vi "Ball at defense area.vi"(10 "IA State":T1) -> (2 "Ball at defense area ?":bool)   [LabVIEW 2016]
uses:
  Core/AI Input.ctl
  Core/AI Robot.ctl
  Intel/Functions Enum.ctl
  Core/AI Ball.ctl
  Core/Field Size.ctl
  Core/AI Judge.ctl
  Intel/Command Enum.ctl
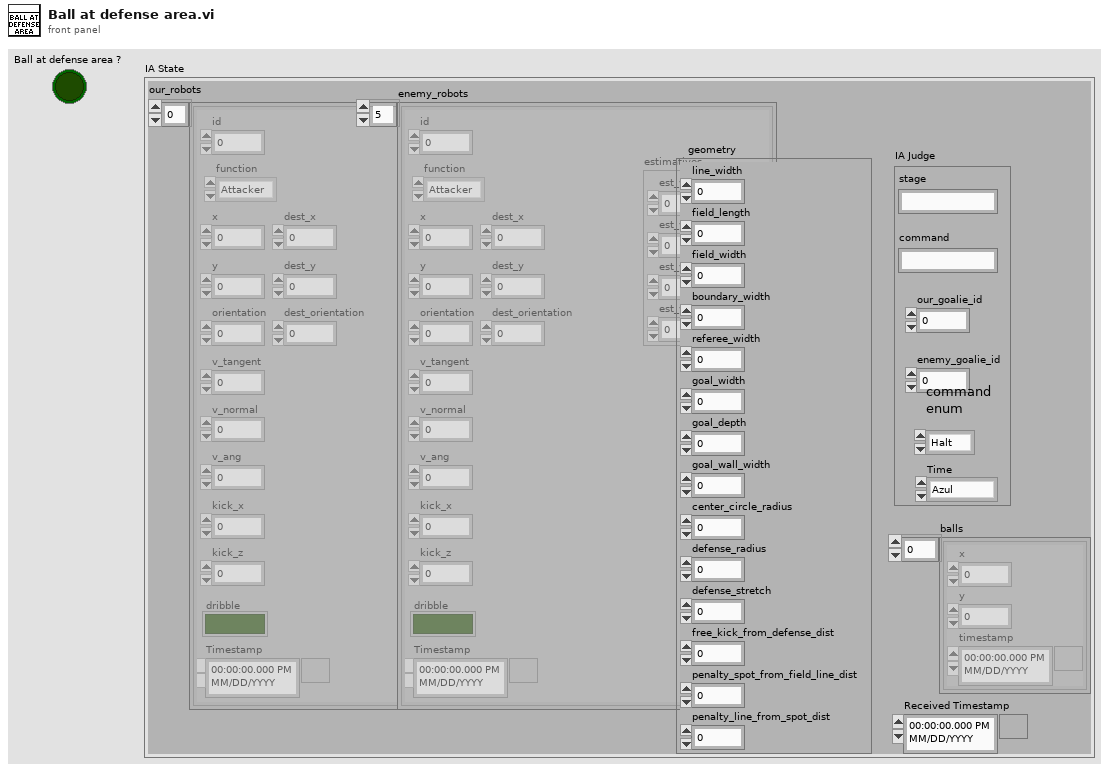
[diagram p1: front panel]
types:
  T1 = typedef "AI Input.ctl" = cluster{"our_robots":T2[], "enemy_robots":T2[], "balls":T4[], "geometry":T5, "IA Judge":T6, "Received Timestamp":timestamp}
  T2 = typedef "AI Robot.ctl" = cluster{"id":u32, "function":T3, "x":dbl, "y":dbl, "orientation":dbl, "v_tangent":dbl, "v_normal":dbl, "v_ang":dbl, "kick_x":dbl, "kick_z":dbl, "dribble":bool, "Timestamp":timestamp, "dest_x":dbl, "dest_y":dbl, "dest_orientation":dbl, "estimatives":cluster{"est_v_tangent":dbl, "est_v_normal":dbl, "est_vx":dbl, "est_vy":dbl}}
  T3 = typedef "Functions Enum.ctl" = enum16{"Attacker", "Goalie", "Defender", "Striker", "Goto 0", "Dummy", "ZigZag"}
  T4 = typedef "AI Ball.ctl" = cluster{"x":dbl, "y":dbl, "timestamp":timestamp}
  T5 = typedef "Field Size.ctl" = cluster{"line_width":u32, "field_length":u32, "field_width":u32, "boundary_width":u32, "referee_width":u32, "goal_width":u32, "goal_depth":u32, "goal_wall_width":u32, "center_circle_radius":u32, "defense_radius":u32, "defense_stretch":u32, "free_kick_from_defense_dist":u32, "penalty_spot_from_field_line_dist":u32, "penalty_line_from_spot_dist":u32}
  T6 = typedef "AI Judge.ctl" = cluster{"stage":string, "command":string, "our_goalie_id":dbl, "enemy_goalie_id":dbl, "command\nenum":T7, "Time":enum16{"Azul", "Amarelo"}}
  T7 = typedef "Command Enum.ctl" = enum16{"Halt", "Stop", "Force Start", "PKA Normal Start", "Prepare Kickoff Ally", "PKE Normal Start", "Prepare Kickoff Enemy", "Prepare Penalty Ally", "PPA Normal Start", "Prepare Penalty Enemy", "PPE Normal Start", "Direct Free Enemy", "Direct Free Ally", "Indirect Free Enemy", "Indirect Free Ally", "Timeout Enemy", "Timeout Ally", "Goal Enemy", "Goal Ally", "Ball Placement Enemy", "Ball Placement Ally", "None"}
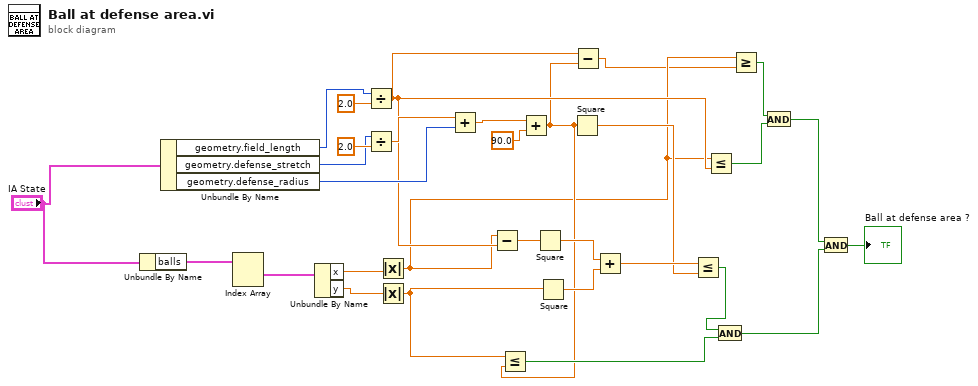
[diagram p0: block diagram]
diagram:
  n1 = Unbundle By Name("IA State") -> ("balls"=w30:T4[])
  n2 = Unbundle By Name("IA State") -> ("geometry.field_length"=w23:u32, "geometry.defense_stretch"=w22:u32, "geometry.defense_radius"=w16:u32)
  n3 = Index Array(array=w30) -> (element #1=w29:T4)  [unwired: 2 in, 1 out]
  n4 = Unbundle By Name(w29) -> ("x"=w26:dbl, "y"=w27:dbl)
  n5 = Divide(x=w23, y=2.0) -> (x/y=w9:dbl)
  n6 = Divide(x=w22, y=2.0) -> (x/y=w17:dbl)
  n7 = Absolute Value(x=w26) -> (abs(x)=w7:dbl)
  n8 = Absolute Value(x=w27) -> (abs(x)=w12:dbl)
  n9 = Add(x=w17, y=w16) -> (x+y=w15:dbl)
  n10 = Subtract(x=w7, y=w9) -> (x-y=w21:dbl)
  n11 = Add(x=w15, y=90.0 ("x")) -> (x+y=w8:dbl)
  n12 = Less Or Equal?(x=w12, y=w8) -> (x <= y?=w11:bool)
  n13 = Square(x=w21) -> (x^2=w20:dbl)
  n14 = Square(x=w12) -> (x^2=w19:dbl)
  n15 = Square(x=w8) -> (x^2=w13:dbl)
  n16 = Subtract(x=w9, y=w8) -> (x-y=w6:dbl)
  n17 = Add(x=w20, y=w19) -> (x+y=w18:dbl)
  n18 = Less Or Equal?(x=w18, y=w13) -> (x <= y?=w10:bool)
  n19 = Less Or Equal?(x=w7, y=w9) -> (x <= y?=w4:bool)
  n20 = And(x=w10, y=w11) -> (x .and. y?=w3:bool)
  n21 = Greater Or Equal?(x=w7, y=w6) -> (x >= y?=w5:bool)
  n22 = And(x=w5, y=w4) -> (x .and. y?=w2:bool)
  n23 = And(x=w2, y=w3) -> (x .and. y?=→"Ball at defense area ?":bool)
